vi "BMP085 Read Temp & Press.vi"(8 "error in (no error)":errorcluster, 11 "BMP085 (GY-65) in":refnum<class "BMP085 (GY-65).lvclass">) -> (0 "error out":errorcluster, 1 "hPa":dbl format="%.1f", 2 "Temp [°C]":dbl format="%.1g", 3 "BMP085 (GY-65) out":refnum<class "BMP085 (GY-65).lvclass">)   [LabVIEW 2015, in "BMP085 (RT).lvlib"]
uses:
  BMP085 (RT).lvlib
  BMP085 (GY-65).lvclass
panel:
  out "UT":i32
  out "UP":i32
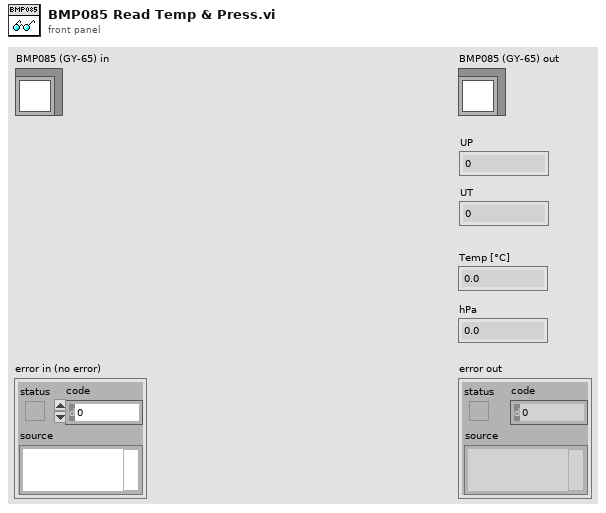
[diagram p1: front panel]
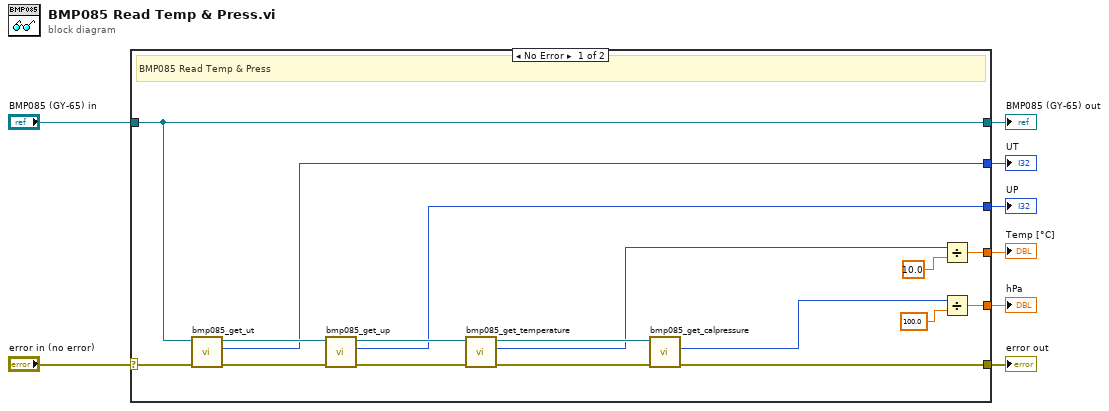
[diagram p0: block diagram]
diagram:
  n1 = case shown="No Error" "error in (no error)" {
    selector: "error in (no error)" -> [w25 w27]
    tunnel: [w21 w27] -> w7
    tunnel: [w20 w26] -> w5
    tunnel: "BMP085 (GY-65) in" -> [w20 w26]
    tunnel: [w14 _] -> w4
    tunnel: [w11 _] -> w3
    tunnel: [w10 _] -> w2
    tunnel: [w9 _] -> w1
    frame No Error {
      # "BMP085 Read Temp & Press"
      n2 = call "bmp085_get_ut.vi"("error in (no error)"=w25, "BMP085 (GY-65) in"=w20) -> ("error out"=w24:errorcluster, "UT"=w9:i32, "BMP085 (GY-65) out"=w19:refnum<class "BMP085 (GY-65).lvclass">)  [unwired: 7 in]
      n3 = call "bmp085_get_up.vi"("error in (no error)"=w24, "BMP085 (GY-65) in"=w19) -> ("error out"=w23:errorcluster, "UP"=w10:i32, "BMP085 (GY-65) out"=w18:refnum<class "BMP085 (GY-65).lvclass">)  [unwired: 7 in]
      n4 = call "bmp085_get_temperature.vi"("error in (no error)"=w23, "BMP085 (GY-65) in"=w18) -> ("error out"=w22:errorcluster, "T"=w15:i32, "BMP085 (GY-65) out"=w17:refnum<class "BMP085 (GY-65).lvclass">)  [unwired: 7 in]
      n5 = call "bmp085_get_calpressure.vi"("error in (no error)"=w22, "BMP085 (GY-65) in"=w17) -> ("error out"=w21:errorcluster, "p"=w13:i32)  [unwired: 7 in, 1 out]
      n6 = Divide(x=w15, y=10.0) -> (x/y=w14:dbl)
      n7 = Divide(x=w13, y=100.0) -> (x/y=w11:dbl)
    }
    frame Error {
    }
  }
  "error out" <- w7
  "BMP085 (GY-65) out" <- w5
  "Temp [°C]" <- w4
  "hPa" <- w3
  "UP" <- w2
  "UT" <- w1
